vi "Encoder.vi"() -> ()   [LabVIEW 2017]
uses:
  <vilib>/MakerHub/LINX/Public/Peripherals/Digital/Digital Read 1 Chan.vi
  <vilib>/MakerHub/LINX/Public/Peripherals/Digital/Digital Read N Chans.vi
  <vilib>/MakerHub/LINX/Private/Local IO/LinxDigitalRead.vi
  <vilib>/MakerHub/LINX/Public/Utilities/Check Channel.vi
  <vilib>/MakerHub/LINX/Public/Utilities/Open Serial.vi
  <vilib>/MakerHub/LINX/Private/Utilties/Generate Error.vi
  <vilib>/MakerHub/LINX/LMH-LINX.lvlib
panel:
  in  "stop":bool
  in  "DI Channel":u8
  in  "Serial Port":refnum<visa-resource-name>="N/A"
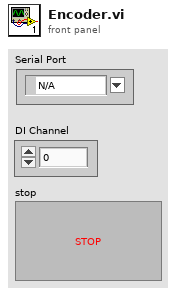
[diagram p1: front panel]
types:
  T1 = typedef "LMH-LINX.lvlib/LINX Ref.ctl" = cluster{"IO":T2, "Interface":T3, "LINX Device Config":T4}
  T2 = typedef "LMH-LINX.lvlib/Platform.ctl" = enum16{"Remote", "Local"}
  T3 = typedef "LMH-LINX.lvlib/Interface.ctl" = enum16{"Serial", "TCP"}
  T4 = typedef "LMH-LINX.lvlib/Device.lvlib/LINX Device Config.ctl" = cluster{"Interface":T3, "COM Port":refnum<visa-resource-name>, "TCP Configuration":T5, "Device Family":u8, "Device ID":u8, "Device Name":string, "TCP Ref":refnum<k5>, "Channels":T6}
  T5 = typedef "LMH-LINX.lvlib/Device.lvlib/TCP Config.ctl" = cluster{"IP Address":string, "Port":u16}
  T6 = typedef "LMH-LINX.lvlib/Channels.ctl" = cluster{"DI":u8[], "DO":u8[], "AI":u8[], "AO":u8[], "PWM":u8[], "QE":u8[], "UART":u8[], "I2C 2":u8[], "SPI":u8[], "CAN":u8[], "Servo":u8[], "AI Ref (V)":dbl, "AI Resolution (Bits)":u8, "AO Ref (V)":dbl, "AO Resolution (Bits)":u8}
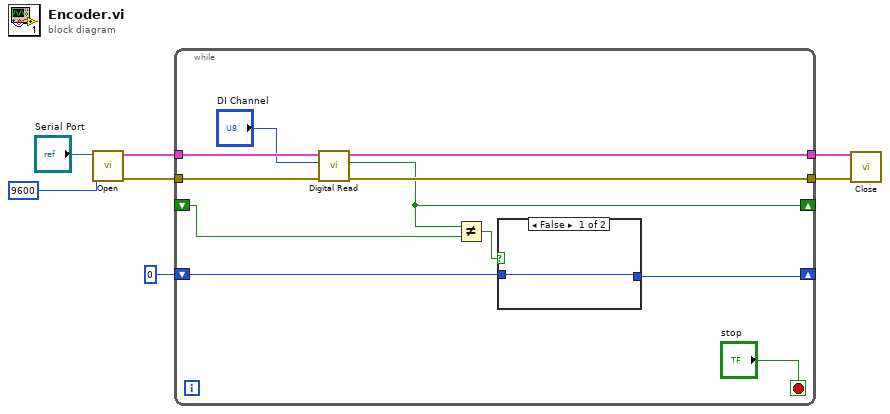
[diagram p0: block diagram]
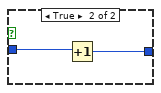
[diagram p2: hidden frame]
diagram:
  n1 = call-poly <vilib>:"Open.vi"("Baud Rate Override"=u32 9600, "Serial Port"="Serial Port") -> ("Error Out"=w3:errorcluster, "LINX Resource"=w7:T1)  [unwired: 7 in, 1 out]
  n2 = while {
    tunnel: w7 -> [w18]
    shift-right: [w12] -> _
    shift-left: _ -> [w13]
    tunnel: [w17] -> w4
    tunnel: w3 -> [w15]
    tunnel: [w14] -> w2
    shift-right: [w9] -> _
    shift-left: 0 -> [w10]
    stop <- "stop" stop-if-true
    n3 = call-poly <vilib>:"Digital Read.vi"("Error In"=w15, "DI Channel"="DI Channel", "LINX Resource"=w18) -> ("Error Out"=w14:errorcluster, "DI Value"=w12:bool, "LINX Resource"=w17:T1)  [unwired: 6 in]
    n4 = Not Equal?(x=w12, y=w13) -> (x != y?=w11:bool)
    n5 = case shown="False" w11 {
      tunnel: w10 -> [w19 w21]
      tunnel: [w19 w20] -> w9
      frame False {
      }
      frame True {
        n6 = Increment(x=w21) -> (x+1=w20:i32)
      }
    }
  }
  n7 = call <vilib>:"Close.vi"("Error In"=w2, "LINX Resource"=w4) -> ()  [unwired: 9 in, 1 out]
